vi "Create_Log_File.vi"(0 "Application_Directory":path) -> (4 "New_File_Path":path)   [LabVIEW 2021]
doc: "Used to create log file Name"
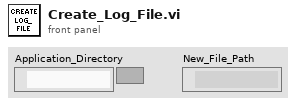
[diagram p1: front panel]
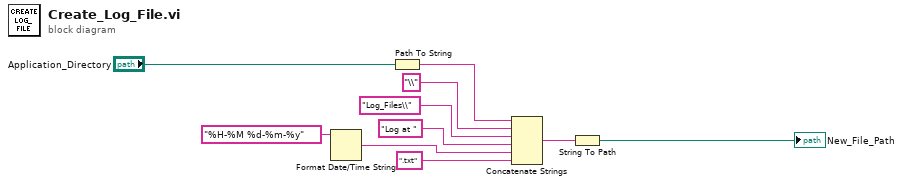
[diagram p0: block diagram]
diagram:
  n1 = Format Date/Time String(time format string (%c)="%H-%M %d-%m-%y") -> (date/time string=w8:string)  [unwired: 2 in]
  n2 = Path To String(path="Application_Directory") -> (string=w7:string)
  n3 = Concatenate Strings(w7, "\\" ("string"), "Log_Files\\" ("string"), "Log at ", w8, ".txt" ("string")) -> (w6:string)
  n4 = String To Path(string=w6) -> (path=→"New_File_Path":path)
